vi "Connect.vi"(8 "error in":errorcluster, 11 "4081 in":refnum<class "4081.lvclass">) -> (0 "error out":errorcluster, 3 "4081 out":refnum<class "4081.lvclass">)   [LabVIEW 2019, in "4081.lvlib" / "4081.lvclass"]
uses:
  Library/4081.lvclass
  C:/Users/Public/Documents/Development/builds/Instruments/Instruments.lvlibp/Library/Instruments.lvclass
  Library/4081.lvclass/4081.ctl
  Accessors/Write Local Resource.vi
  builds/Instruments/Instruments.lvlibp/Accessors/Read Resource.vi
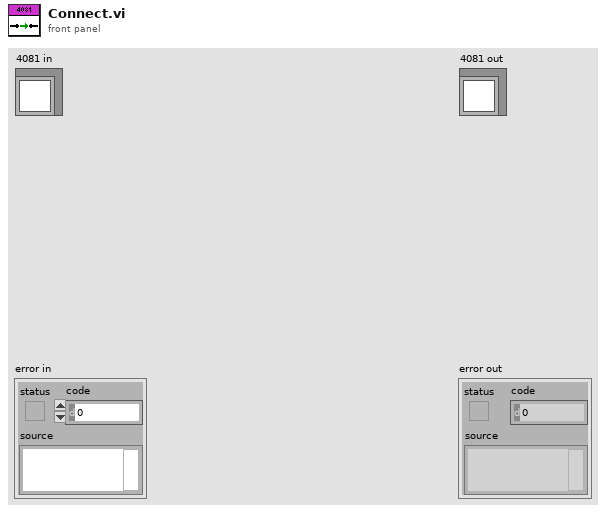
[diagram p1: front panel]
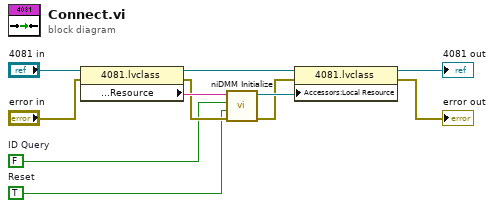
[diagram p0: block diagram]
diagram:
  w1 = TRUE  # Reset
  w2 = FALSE  # ID Query
  n1 = property class="4081.lvclass"(reference="4081 in", error in="error in") -> (reference out=w7:refnum<class "4081.lvclass">, error out=w6:errorcluster, "Accessors:Configuration:Resource"=w9:string)
  n2 = call <instrlib>:"niDMM Initialize.vi"("error in (no error)"=w6, "Reset"=w1, "ID Query"=w2, "Instrument Descriptor"=w9) -> ("error out"=w5:errorcluster, "instrument handle out"=w8:refnum<k15>)  [unwired: 6 in]
  n3 = property class="4081.lvclass"(reference=w7, error in=w5, "Accessors:Local Resource"=w8) -> (reference out=→"4081 out":refnum<class "4081.lvclass">, error out=→"error out":errorcluster)
